vi "sensor array to indices.vi"(11 "Sensor Array":T1) -> (3 "Channel Indices":i32[](array[numeric]))   [LabVIEW 2010]
uses:
  channel identifier.ctl
  Sensor array.ctl
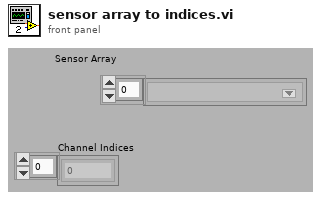
[diagram p1: front panel]
types:
  T1 = typedef "Sensor array.ctl" = T2[]
  T2 = typedef "channel identifier.ctl" = u16
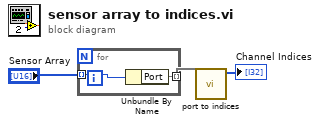
[diagram p0: block diagram]
diagram:
  n1 = for {
    tunnel: "Sensor Array" -> [w5] mode=indexing
    tunnel: [w4] -> w2 mode=indexing
    n2 = Unbundle By Name(w5) -> ("Port"=w4)
  }
  n3 = call "port to indices.vi"("Port"=w2) -> ("Channel Indices"=→"Channel Indices":i32[])  [unwired: 10 in]
